vi "SerialCOM.vi"(1 "Function":T1(ring), 5 "byte count":u32, 7 "write buffer":string, 9 "ReadDelay (s)":dbl caption="Delay Time (s)", 11 "error in (no error)":errorcluster, 12 "Port Setting":T2={"baud rate"=9600, "data bits"=8, "parity (0:none)"=enum."None", "stop bits (10: 1 bit)"=10} {"stop bits (10: 1 bit)" items=["1.0"=10, "1.5"=15, "2.0"=20]; "data bits" min=5 max=8 step=1}, 13 "VISA_IN":refnum<visa-resource-name>) -> (3 "Success?":bool, 4 "return count":u32, 6 "Read Buffer":string, 8 "array Out":u8[](array[numeric]), 10 "Bytes at Port":u32, 15 "error out":errorcluster)   [LabVIEW 2014]
uses:
  <vilib>/Instr/_visa.llb/VISA Flush IO Buffer Mask.ctl
  <vilib>/Instr/_visa.llb/VISA Configure Serial Port (Instr).vi
panel:
  out "VISA _OUT":refnum<visa-resource-name>
  # "IN"
  # "OUT"
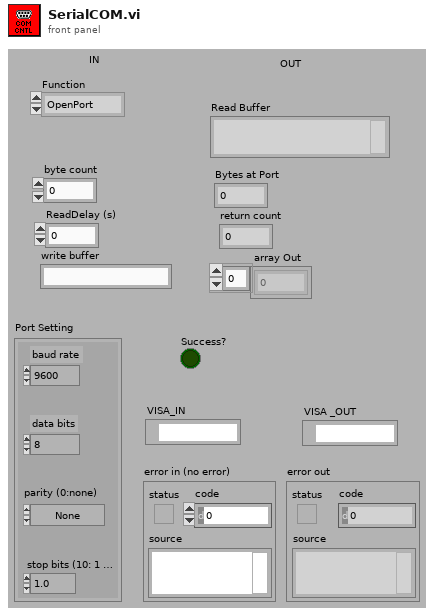
[diagram p1: front panel]
types:
  T1 = enum16{"OpenPort", "Initial Serial Port", "Write", "ByteRead", "Read", "ClearBuff", "Close"}
  T2 = cluster{"baud rate":u32, "data bits":u16, "parity (0:none)":enum16{"None", "Odd", "Even", "Mark", "Space"}, "stop bits (10: 1 bit)":u16}
  T3 = typedef "VISA Flush IO Buffer Mask.ctl" = u16
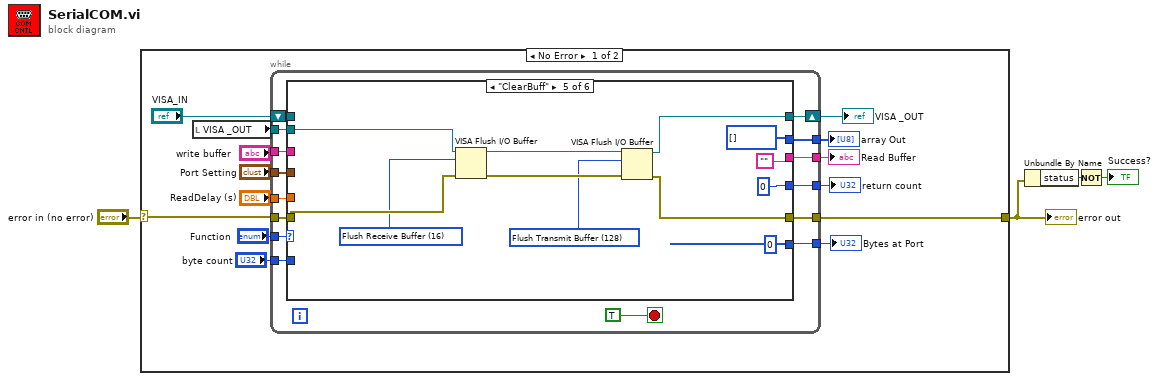
[diagram p0: block diagram]
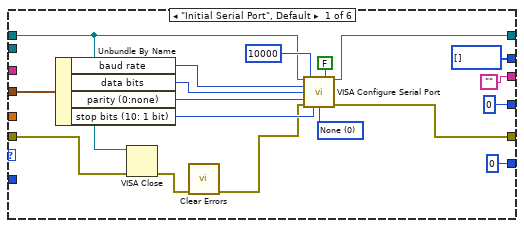
[diagram p2: hidden frame]
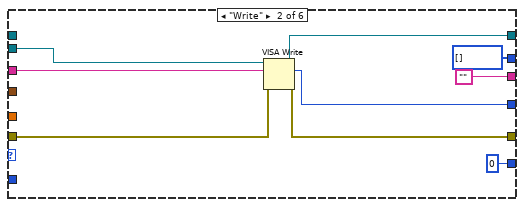
[diagram p3: hidden frame]
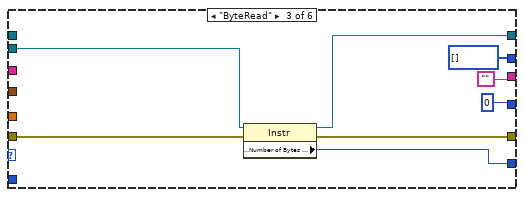
[diagram p4: hidden frame]
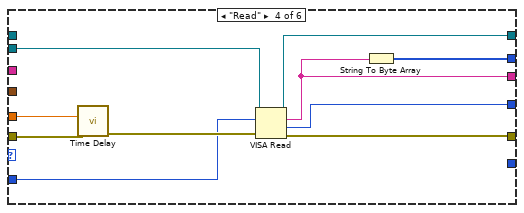
[diagram p5: hidden frame]
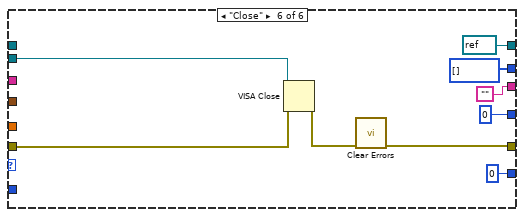
[diagram p6: hidden frame]
diagram:
  n1 = case shown="No Error" "error in (no error)" {
    selector: "error in (no error)" -> [w8 w100]
    tunnel: [w11 w100] -> w3
    frame No Error {
      n2 = local read "VISA _OUT"() -> (w5:refnum<visa-resource-name>)
      n3 = while {
        tunnel: "Function" -> [w33]
        tunnel: "Port Setting" -> [w32]
        tunnel: w8 -> [w31]
        tunnel: "write buffer" -> [w30]
        tunnel: [w29] -> w13
        tunnel: [w28] -> w11
        tunnel: [w27] -> w12
        tunnel: "ReadDelay (s)" -> [w26]
        tunnel: [w24] -> w14
        tunnel: [w23] -> w10
        tunnel: "byte count" -> [w22]
        shift-right: [w21] -> w6
        shift-left: "VISA_IN" -> [w20]
        tunnel: w5 -> [w19]
        stop <- TRUE stop-if-true
        n4 = case shown="\"ClearBuff\"" w33 {
          tunnel: w20 -> [w36 _ _ _ _ _]
          tunnel: w32 -> [w51 _ _ _ _ _]
          tunnel: w31 -> [w37 w60 w68 w77 w86 w99]
          tunnel: [w40 w58 w67 w72 w87 w93] -> w28
          tunnel: w30 -> [_ w59 _ _ _ _]
          tunnel: ["" "" "" w75 "" ""] -> w29
          tunnel: [w41 w56 w65 w78 w85 refnum<visa-resource-name> refnum ("VISA resource name")] -> w21
          tunnel: [u32 0 ("return count") w55 u32 0 ("Bytes at Port") w73 u32 0 ("return count") u32 0 ("return count")] -> w27
          tunnel: w26 -> [_ _ _ w76 _ _]
          tunnel: [u8[] [] ("unsigned byte array") u8[] [] ("unsigned byte array") u8[] [] ("unsigned byte array") w74 u8[] [] ("unsigned byte array") u8[] [] ("unsigned byte array")] -> w24
          tunnel: [u32 0 ("Bytes at Port") u32 0 ("Bytes at Port") w66 _ u32 0 ("Bytes at Port") u32 0 ("Bytes at Port")] -> w23
          tunnel: w22 -> [_ _ _ w70 _ _]
          tunnel: w19 -> [_ w52 w61 w69 w79 w91]
          frame "Initial Serial Port", Default {
            w42 = u16 0 items=["None", "XON/XOFF", "RTS/CTS", "XON/XOFF & RTS/CTS", "DTR/DSR", "XON/XOFF & DTR/DSR"] ("flow control (0:none)")
            n5 = Unbundle By Name(w51) -> ("baud rate"=w50:u32, "data bits"=w49:u16, "parity (0:none)"=w48:enum16{"None", "Odd", "Even", "Mark", "Space"}, "stop bits (10: 1 bit)"=w47:u16)
            n6 = VISA Close(VISA resource name=w36, error in (no error)=w37) -> (error out=w35:errorcluster)
            n7 = call <vilib>:"Clear Errors.vi"("error in (no error)"=w35) -> ("error out"=w34:errorcluster)  [unwired: 5 in, 1 out]
            n8 = call-poly "VISA Configure Serial Port"("VISA resource name"=w36, "timeout (10sec)"=u32 10000, "Enable Termination\nChar (T)"=FALSE ("Enable Termination\nChar (T)"), "baud rate (9600)"=w50, "data bits (8)"=w49, "parity (0:none)"=w48, "error in (no error)"=w34, "stop bits (10: 1 bit)"=w47, "flow control (0:none)"=w42) -> ("VISA resource name out"=w41:refnum<visa-resource-name>, "error out"=w40:errorcluster)  [unwired: 5 in]
          }
          frame "Write" {
            n9 = VISA Write(VISA resource name=w52, write buffer=w59, error in (no error)=w60) -> (VISA resource name out=w56:refnum<visa-resource-name>, return count=w55:u32, error out=w58:errorcluster)
          }
          frame "ByteRead" {
            n10 = property class="Instr"(reference=w61, error in=w68) -> (reference out=w65:refnum<visa-resource-name>, error out=w67:errorcluster, "Serial Settings:Number of Bytes at Serial Port"=w66:u32)
          }
          frame "Read" {
            n11 = call "Time Delay"("error in (no error)"=w77, "Delay Time (s)"=w76) -> ("error out"=w71:errorcluster)  [unwired: 9 in]
            n12 = VISA Read(VISA resource name=w69, byte count=w70, error in (no error)=w71) -> (VISA resource name out=w78:refnum<visa-resource-name>, read buffer=w75:string, return count=w73:u32, error out=w72:errorcluster)
            n13 = String To Byte Array(string=w75) -> (unsigned byte array=w74:u8[])
          }
          frame "ClearBuff" {
            w83 = T3 128 items=["Flush Receive Buffer"=16, "Write Transmit Buffer to Device"=32, "Flush Receive Buffer (No I/O)"=64, "Flush Transmit Buffer"=128] ("Mask")
            w84 = T3 16 items=["Flush Receive Buffer"=16, "Write Transmit Buffer to Device"=32, "Flush Receive Buffer (No I/O)"=64, "Flush Transmit Buffer"=128] ("Mask")
            n14 = VISA Flush I/O Buffer(VISA resource name=w79, mask (16)=w84, error in (no error)=w86) -> (VISA resource name out=w89:refnum<visa-resource-name>, error out=w88:errorcluster)
            n15 = VISA Flush I/O Buffer(VISA resource name=w89, mask (16)=w83, error in (no error)=w88) -> (VISA resource name out=w85:refnum<visa-resource-name>, error out=w87:errorcluster)
          }
          frame "Close" {
            n16 = VISA Close(VISA resource name=w91, error in (no error)=w99) -> (error out=w94:errorcluster)
            n17 = call <vilib>:"Clear Errors.vi"("error in (no error)"=w94) -> ("error out"=w93:errorcluster)  [unwired: 5 in, 1 out]
          }
        }
      }
      "Read Buffer" <- w13
      "VISA _OUT" <- w6
      "return count" <- w12
      "array Out" <- w14
      "Bytes at Port" <- w10
    }
    frame Error {
    }
  }
  "error out" <- w3
  n18 = Unbundle By Name(w3) -> ("status"=w2:bool)
  n19 = Not(x=w2) -> (.not. x?=→"Success?":bool)
